vi "Subscr.Subscribe to Event.vi"(4 "Disable":bool, 6 "Source Q":refnum<queue>, 7 "Source Q Name":string, 8 "error in (no error)":errorcluster, 9 "Data Element":T1, 10 "Event Name":string, 11 "Local Q":refnum<queue>) -> (0 "error out":errorcluster, 3 "Local Q Dup":refnum<queue>)   [LabVIEW 2024, in "EQMF.lvlib" / "Subscription.lvlib" / "Subscription.lvclass"]
uses:
  Subscription.lvclass
  Queues/Q.Element.ctl
  Subscr.Subscription Request Info.ctl
  Queues/Queue Utils.lvlib
  Subscription.lvlib
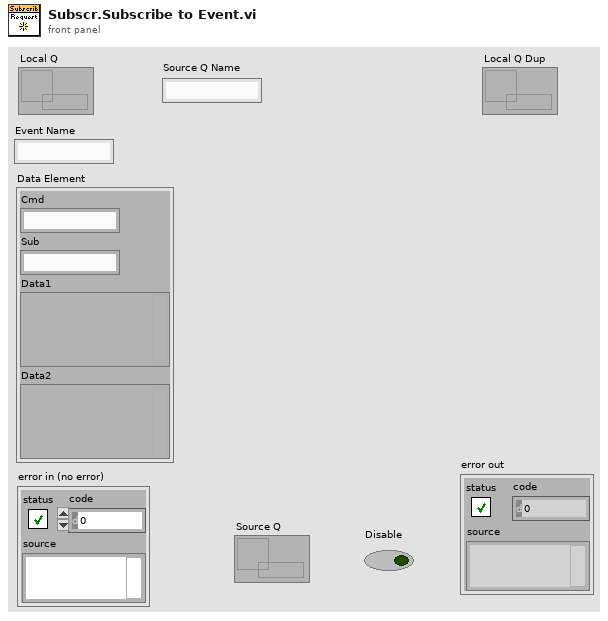
[diagram p1: front panel]
types:
  T1 = typedef "EQMF.lvlib/Queue Utils.lvlib/Q.Element.ctl" = cluster{"Cmd":string, "Sub":string, "Data1":variant, "Data2":variant}
  T2 = typedef "EQMF.lvlib/Subscription.lvlib/Subscr.Subscription Request Info.ctl" = cluster{"Name":string, "Data Q":refnum<queue>, "Data Element":T1}
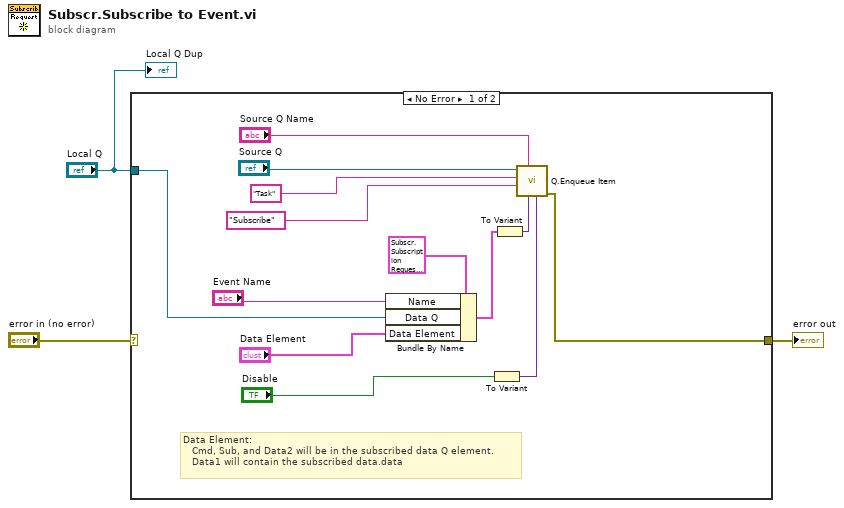
[diagram p0: block diagram]
diagram:
  n1 = case shown="No Error" "error in (no error)" {
    selector: "error in (no error)" -> [_ w17]
    tunnel: [w15 w17] -> w2
    tunnel: "Local Q" -> [w10 _]
    frame No Error {
      # "Data Element:  \n   Cmd, Sub, and Data2 will be in the subscribed data Q element.\n   Data1 will contain the subscribed data.data"
      n2 = Bundle By Name(cluster=T2 {"Name"="", "Data Q"=refnum, "Data Element"={"Cmd"="", "Sub"="", "Data1"=variant, "Data2"=variant}} ("Event Destination"), "Name"="Event Name", "Data Q"=w10, "Data Element"="Data Element") -> (w8:T2)
      n3 = To Variant(anything="Disable") -> (Variant=w6:variant)
      n4 = To Variant(anything=w8) -> (Variant=w13:variant)
      n5 = call "Q.Enqueue Item.vi"("Data2"=w6, "Data1"=w13, "Q Name"="Source Q Name", "Sub"="Subscribe" ("Cmd"), "Cmd"="Task", "Q In"="Source Q") -> ("error out"=w15:errorcluster)  [unwired: 4 in, 1 out]
    }
    frame Error {
    }
  }
  "error out" <- w2
  "Local Q Dup" <- "Local Q"
